vi "Parse Data to Variant with Type Information.vi"(8 "error in (no error)":errorcluster, 10 "Data":string, 11 "Datatype":string) -> (0 "error out":errorcluster, 3 "Variant":variant)   [LabVIEW 2020, in "LUnit Test Vector.lvclass"]
uses:
  LUnit Test Vector.lvclass
  <vilib>/Utility/Data Type/Type Definitions/Data Type.ctl
  <vilib>/Utility/error.llb/Error Cluster From Error Code.vi
  <vilib>/ErrorRing/Error Ring.xnode
  <vilib>/Utility/Data Type/NI_Data Type.lvlib
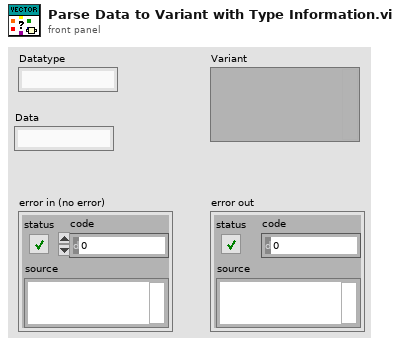
[diagram p1: front panel]
types:
  T1 = typedef "NI_Data Type.lvlib/Data Type.ctl" = enum8{"Invalid Type", "Void", "I8", "I16", "I32", "I64", "U8", "U16", "U32", "U64", "Single Float", "Double Float", "Extended Float", "Single Complex", "Double Complex", "Extended Complex", "Enum U8", "Enum U16", "Enum U32", "Enum U64", "Single Float With Unit", "Double Float With Unit", "Extended Float With Unit", "Single Complex with Unit", "Double Complex with Unit", "Extended Complex with Unit", "Boolean", "String", "Path", "Picture", "Tag", "Array", "Cluster", "Variant", "LV Variant", "Waveform", "Timestamp", "Digital Waveform", "Digital Data", "ExpressData", "Refnum", "External Data", "VI", "Poly VI", "LabVIEW Class Instance", "Fixed Point", "Set Collection", "Map Collection"}
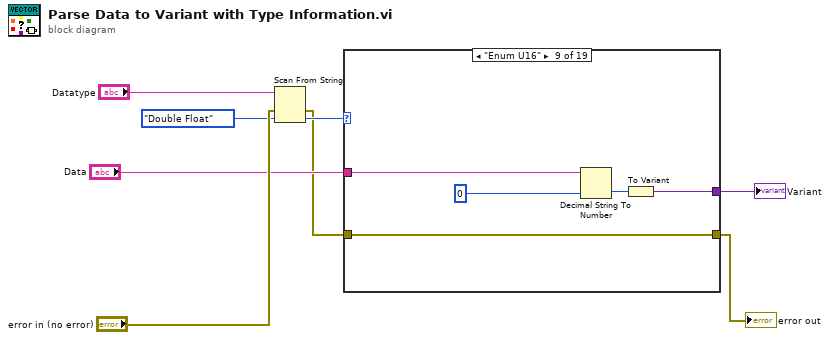
[diagram p0: block diagram]
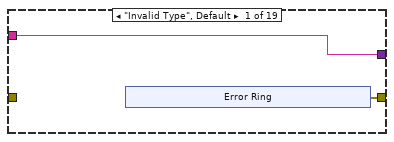
[diagram p2: hidden frame]
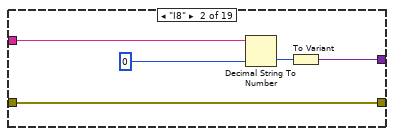
[diagram p3: hidden frame]
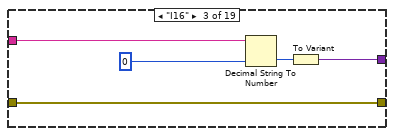
[diagram p4: hidden frame]
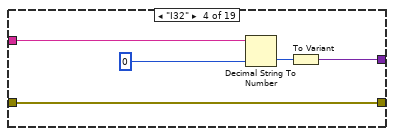
[diagram p5: hidden frame]
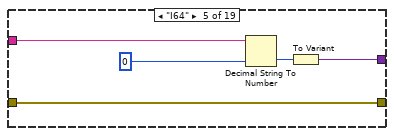
[diagram p6: hidden frame]
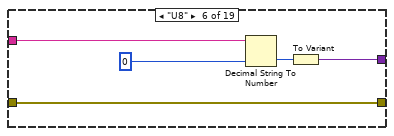
[diagram p7: hidden frame]
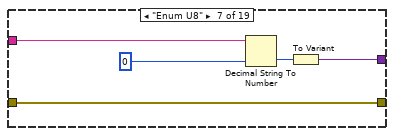
[diagram p8: hidden frame]
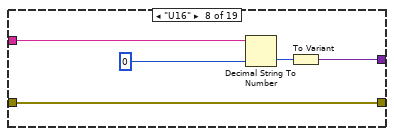
[diagram p9: hidden frame]
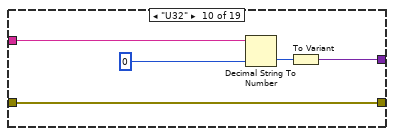
[diagram p10: hidden frame]
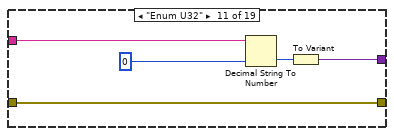
[diagram p11: hidden frame]
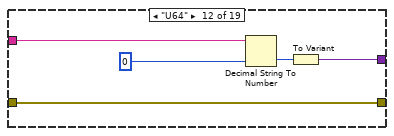
[diagram p12: hidden frame]
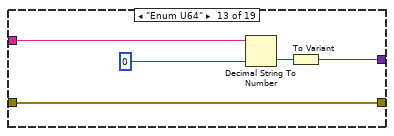
[diagram p13: hidden frame]
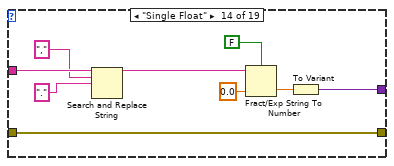
[diagram p14: hidden frame]
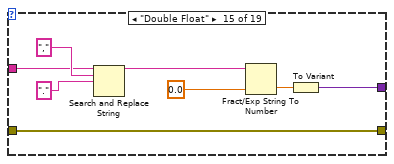
[diagram p15: hidden frame]
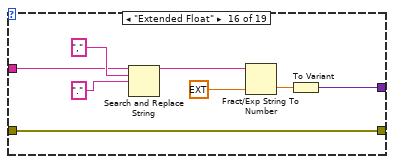
[diagram p16: hidden frame]
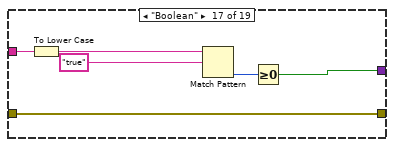
[diagram p17: hidden frame]
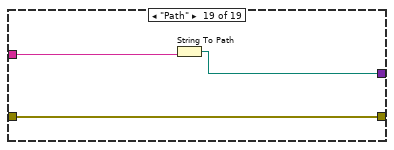
[diagram p19: hidden frame]
diagram:
  n1 = Scan From String(input string="Datatype", error in="error in (no error)", default 1=Data_Type."Double Float" ("type")) -> (error out=w1:errorcluster, output 1=w5:T1)  [unwired: 2 in, 2 out]
  n2 = case shown="\"Enum U16\"" w5 {
    tunnel: "Data" -> [w10 w19 w24 w29 w34 w39 w44 w49 w54 w59 w64 w69 w74 w78 w84 w93 w105 w107 w110]
    tunnel: [w10 w16 w21 w26 w31 w36 w41 w46 w51 w56 w61 w66 w71 w81 w89 w97 w101 w107 w109] -> w3
    tunnel: [w9 w15 w20 w25 w30 w35 w40 w45 w50 w55 w60 w65 w70 w80 w88 w96 w100 w106 w108] -> w2
    tunnel: w1 -> [_ w15 w20 w25 w30 w35 w40 w45 w50 w55 w60 w65 w70 w80 w88 w96 w100 w106 w108]
    frame "Invalid Type", Default {
      n3 = xnode "Error Ring"() -> ("error out"=w9:errorcluster)
    }
    frame "I8" {
      n4 = Decimal String To Number(string=w19, default (0L)=i8 0 ("default (0 I32)")) -> (number=w17:i8)  [unwired: 1 in, 1 out]
      n5 = To Variant(anything=w17) -> (Variant=w16:variant)
    }
    frame "I16" {
      n6 = Decimal String To Number(string=w24, default (0L)=i16 0 ("default (0 I32)")) -> (number=w22:i16)  [unwired: 1 in, 1 out]
      n7 = To Variant(anything=w22) -> (Variant=w21:variant)
    }
    frame "I32" {
      n8 = Decimal String To Number(string=w29, default (0L)=0 ("default (0 I32)")) -> (number=w27:i32)  [unwired: 1 in, 1 out]
      n9 = To Variant(anything=w27) -> (Variant=w26:variant)
    }
    frame "I64" {
      n10 = Decimal String To Number(string=w34, default (0L)=i64 0 ("default (0 I32)")) -> (number=w32:i64)  [unwired: 1 in, 1 out]
      n11 = To Variant(anything=w32) -> (Variant=w31:variant)
    }
    frame "U8" {
      n12 = Decimal String To Number(string=w39, default (0L)=u8 0 ("default (0 I32)")) -> (number=w37:u8)  [unwired: 1 in, 1 out]
      n13 = To Variant(anything=w37) -> (Variant=w36:variant)
    }
    frame "Enum U8" {
      n14 = Decimal String To Number(string=w44, default (0L)=u8 0 ("default (0 I32)")) -> (number=w42:u8)  [unwired: 1 in, 1 out]
      n15 = To Variant(anything=w42) -> (Variant=w41:variant)
    }
    frame "U16" {
      n16 = Decimal String To Number(string=w49, default (0L)=u16 0 ("default (0 I32)")) -> (number=w47:u16)  [unwired: 1 in, 1 out]
      n17 = To Variant(anything=w47) -> (Variant=w46:variant)
    }
    frame "Enum U16" {
      n18 = Decimal String To Number(string=w54, default (0L)=u16 0 ("default (0 I32)")) -> (number=w52:u16)  [unwired: 1 in, 1 out]
      n19 = To Variant(anything=w52) -> (Variant=w51:variant)
    }
    frame "U32" {
      n20 = Decimal String To Number(string=w59, default (0L)=u32 0 ("default (0 I32)")) -> (number=w57:u32)  [unwired: 1 in, 1 out]
      n21 = To Variant(anything=w57) -> (Variant=w56:variant)
    }
    frame "Enum U32" {
      n22 = Decimal String To Number(string=w64, default (0L)=u32 0 ("default (0 I32)")) -> (number=w62:u32)  [unwired: 1 in, 1 out]
      n23 = To Variant(anything=w62) -> (Variant=w61:variant)
    }
    frame "U64" {
      n24 = Decimal String To Number(string=w69, default (0L)=u64 0 ("default (0 I32)")) -> (number=w67:u64)  [unwired: 1 in, 1 out]
      n25 = To Variant(anything=w67) -> (Variant=w66:variant)
    }
    frame "Enum U64" {
      n26 = Decimal String To Number(string=w74, default (0L)=u64 0 ("default (0 I32)")) -> (number=w72:u64)  [unwired: 1 in, 1 out]
      n27 = To Variant(anything=w72) -> (Variant=w71:variant)
    }
    frame "Single Float" {
      n28 = Search and Replace String(input string=w78, search string=",", replace string="." ("search string")) -> (result string=w75:string)  [unwired: 5 in, 3 out]
      n29 = Fract/Exp String To Number(use system decimal point (T)=FALSE, string=w75, default (0 dbl)=sgl 0.0 ("default (0 I32)")) -> (number=w82:sgl)  [unwired: 1 in, 1 out]
      n30 = To Variant(anything=w82) -> (Variant=w81:variant)
    }
    frame "Double Float" {
      n31 = Search and Replace String(input string=w84, search string=",", replace string="." ("search string")) -> (result string=w85:string)  [unwired: 5 in, 3 out]
      n32 = Fract/Exp String To Number(string=w85, default (0 dbl)=0.0 ("default (0 I32)")) -> (number=w90:dbl)  [unwired: 2 in, 1 out]
      n33 = To Variant(anything=w90) -> (Variant=w89:variant)
    }
    frame "Extended Float" {
      n34 = Search and Replace String(input string=w93, search string=",", replace string="." ("search string")) -> (result string=w92:string)  [unwired: 5 in, 3 out]
      n35 = Fract/Exp String To Number(string=w92, default (0 dbl)=ext 0.0 ("default (0 I32)")) -> (number=w98:ext)  [unwired: 2 in, 1 out]
      n36 = To Variant(anything=w98) -> (Variant=w97:variant)
    }
    frame "Boolean" {
      n37 = To Lower Case(string=w105) -> (all lower case string=w104:string)
      n38 = Match Pattern(string=w104, regular expression="true") -> (offset past match=w102:i32)  [unwired: 1 in, 3 out]
      n39 = Greater Or Equal To 0?(x=w102) -> (x >= 0?=w101:bool)
    }
    frame "String" {
    }
    frame "Path" {
      n40 = String To Path(string=w110) -> (path=w109:path)
    }
  }
  "error out" <- w2
  "Variant" <- w3
